vi "Create Parameterized Executive.vi"(4 "File Name":string, 6 "Folder":path, 7 "Attribute Name Blacklist":string[](array[string]), 8 "error in (no error)":errorcluster, 9 "Persistence in":refnum<class "IPersist.lvclass">, 10 "Test Executive":refnum<class "ITest Executive.lvclass">, 11 "Test Executive in":refnum<class "Test Executive.lvclass">) -> (0 "error out":errorcluster, 3 "Test Executive out":refnum<class "Test Executive.lvclass">)   [LabVIEW 2017, in "Test Executive.lvlib" / "Test Executive.lvclass"]
uses:
  <vilib>/gpm_packages/@cs/test-executive/Source/Test Executive/TestExecutive/Test Executive.lvclass
  <vilib>/gpm_packages/@cs/test-executive/Source/Test Executive/ITestExecutive/ITest Executive.lvclass
  <vilib>/gpm_packages/@cs/persistence/source/IPersist/IPersist.lvclass
  35263a14-d3f6-459e-9dbf-1f0ba213c23b.vi
  <vilib>/Utility/error.llb/Error Cluster From Error Code.vi
  <vilib>/gpm_packages/@cs/test-executive/Source/Test Executive/TestExecutive Ref/TestExecutive Ref.lvclass
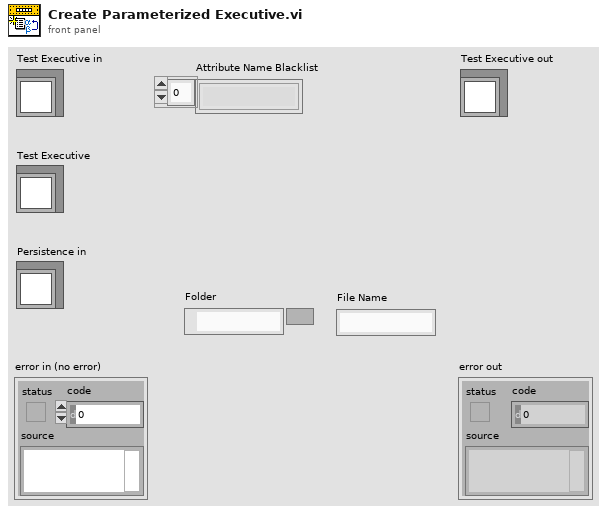
[diagram p1: front panel]
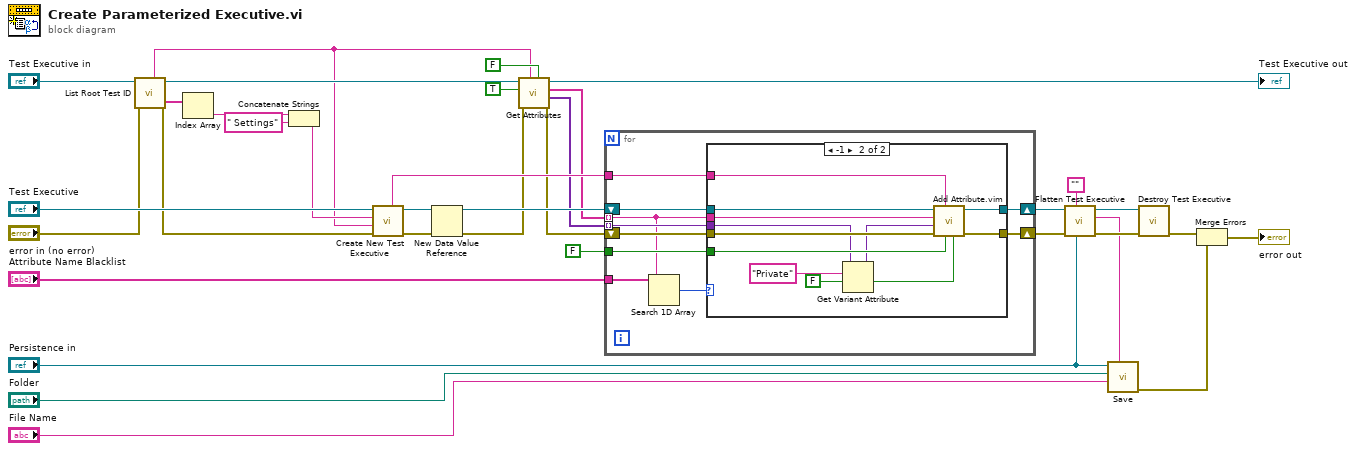
[diagram p0: block diagram]
diagram:
  n1 = call-dynamic "List Root Test ID.vi"("error in (no error)"="error in (no error)", "Test Executive in"="Test Executive in") -> ("error out"=w11:errorcluster, "Test Executive out"=w31:refnum<class "Test Executive.lvclass">, "Root ID"=w19:string, "Root Names"=w26:string[])  [unwired: 5 in, 1 out]
  n2 = Index Array(array=w26) -> (element=w25:string)  [unwired: 1 in]
  n3 = Concatenate Strings(w25, " Settings" ("string")) -> (w23:string)
  n4 = call-dynamic "Create New Test Executive.vi"("error in (no error)"=w11, "Linked List ID"=w19, "Name"=w23, "ITest Executive in"="Test Executive") -> ("error out"=w34:errorcluster, "ITest Executive out"=w35:refnum<class "ITest Executive.lvclass">, "Unique ID out"=w22:string)  [unwired: 5 in]
  n5 = New Data Value Reference(data value=w35, error in=w34) -> (data value reference=w27:refnum<data-value>, error out=w10:errorcluster)
  n6 = call-dynamic "Get Attributes.vi"("Flatten Pointer?"=FALSE, "Test ID"=w19, "error in (no error)"=w10, "Include Private?"=TRUE, "Test Executive in"=w31) -> ("error out"=w9:errorcluster, "Attributes"=w21:variant[], "Attribute Names out"=w20:string[], "Test Executive out"=→"Test Executive out":refnum<class "Test Executive.lvclass">)  [unwired: 1 in, 2 out]
  n7 = for {
    tunnel: w22 -> [w43]
    shift-right: [w45] -> w17
    shift-left: w9 -> [w42]
    shift-right: [w41] -> w16
    shift-left: w27 -> [w44]
    tunnel: w21 -> [w40] mode=indexing
    tunnel: w20 -> [w36] mode=indexing
    tunnel: FALSE -> [w39]
    tunnel: "Attribute Name Blacklist" -> [w37]
    n8 = Search 1D Array(1D array=w37, element=w36) -> (index of element=w38:i32)  [unwired: 1 in]
    n9 = case shown="-1" w38 {
      tunnel: [w46 w59] -> w45
      tunnel: w44 -> [w47 w58]
      tunnel: w43 -> [_ w57]
      tunnel: w42 -> [w46 w56]
      tunnel: [w47 w55] -> w41
      tunnel: w40 -> [_ w50]
      tunnel: w39 -> [_ w54]
      tunnel: w36 -> [_ w53]
      frame Default {
      }
      frame -1 {
        n10 = Get Variant Attribute(Variant=w50, name="Private", default value (empty Variant)=FALSE) -> (duplicate Variant=w49:variant, value=w48:bool)  [unwired: 1 in, 2 out]
        n11 = call "Add Attribute.vim"("Private?"=w48, "Pointer?"=w54, "ID"=w57, "error in (no error)"=w56, "Attribute"=w49, "Attribute Name"=w53, "Test Executive Ref"=w58) -> ("error out"=w59:errorcluster, "Test Executive Ref out"=w55:refnum<data-value>)  [unwired: 1 in, 2 out]
      }
    }
  }
  n12 = call <vilib>:"Flatten Test Executive.vi"("Persistence in"="Persistence in", "Root ID"="", "error in (no error)"=w17, "Test Executive Ref"=w16) -> ("error out"=w15:errorcluster, "Flattened Test Executive"=w6:string, "Test Executive Ref out"=w13:refnum<data-value>)  [unwired: 5 in]
  n13 = call-dynamic "Save.vi"("Flattened String"=w6, "File Name"="File Name", "Folder"="Folder", "IPersist in"="Persistence in") -> ("error out"=w4:errorcluster)  [unwired: 6 in, 1 out]
  n14 = call <vilib>:"Destroy Test Executive.vi"("error in (no error)"=w15, "Test Executive Ref"=w13) -> ("error out"=w14:errorcluster)  [unwired: 9 in]
  n15 = Merge Errors(w14, w4) -> (→"error out":errorcluster)
